vi "setStatus.vi"(8 "error in (no error)":errorcluster, 10 "Status":string, 11 "AndorIKonTempController.lvclass in":refnum<class "AndorIKonTempController.lvclass">) -> (0 "error out":errorcluster, 3 "AndorIKonTempController.lvclass out":refnum<class "AndorIKonTempController.lvclass">)   [LabVIEW 2011, in "Hardware.lvlib" / "Channels.lvlib" / "AndorIKonTempController.lvclass"]
uses:
  AndorIKonTempController.lvclass
  AndorIKonTempController.lvclass/AndorIKonTempController.ctl
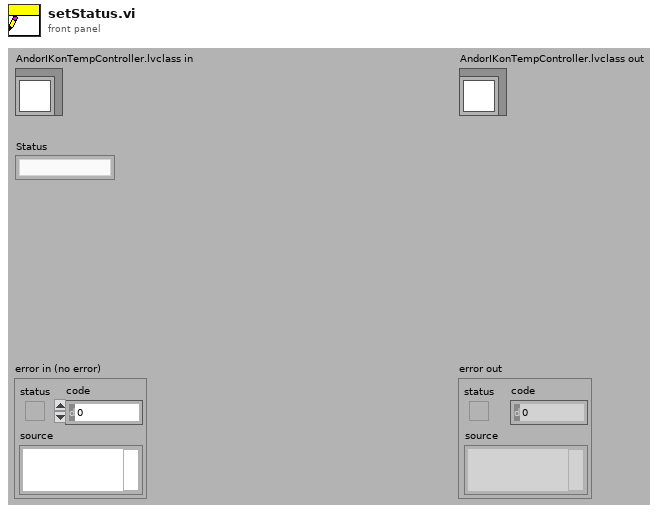
[diagram p1: front panel]
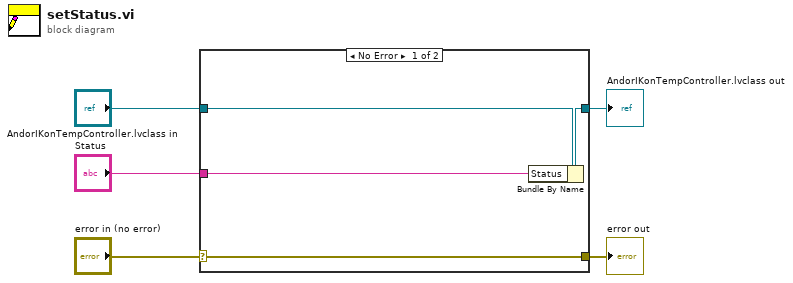
[diagram p0: block diagram]
diagram:
  n1 = case shown="No Error" "error in (no error)" {
    selector: "error in (no error)" -> [w9 w10]
    tunnel: [w9 w10] -> w4
    tunnel: [w7 w11] -> w2
    tunnel: "AndorIKonTempController.lvclass in" -> [w8 w11]
    tunnel: "Status" -> [w6 _]
    frame No Error {
      n2 = Bundle By Name(cluster=w8, "Status"=w6) -> (w7:refnum<class "AndorIKonTempController.lvclass">)
    }
    frame Error {
    }
  }
  "error out" <- w4
  "AndorIKonTempController.lvclass out" <- w2
